vi "Open scan DB HOR.vi"(0 "dup path":path, 5 "Bytes":i64, 7 "Crop top":i32, 9 "Crop bottom":dbl, 11 "Start wavelength":dbl, 12 "End wavelength":dbl, 13 "gap":i32) -> (3 "Bytes done":i64, 4 "Intensity":sgl[](array[numeric]), 15 "wavelengths":sgl[](array[numeric]))   [LabVIEW 2014]
panel:
  # "I havn't a clue \nwhy I thought\nI needed this\nbut it breaks if\nI take it away"
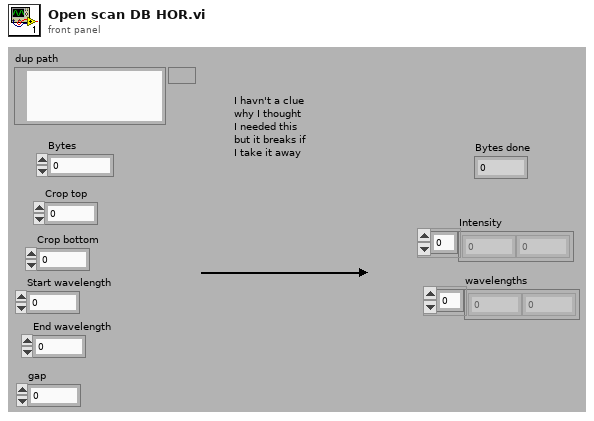
[diagram p1: front panel]
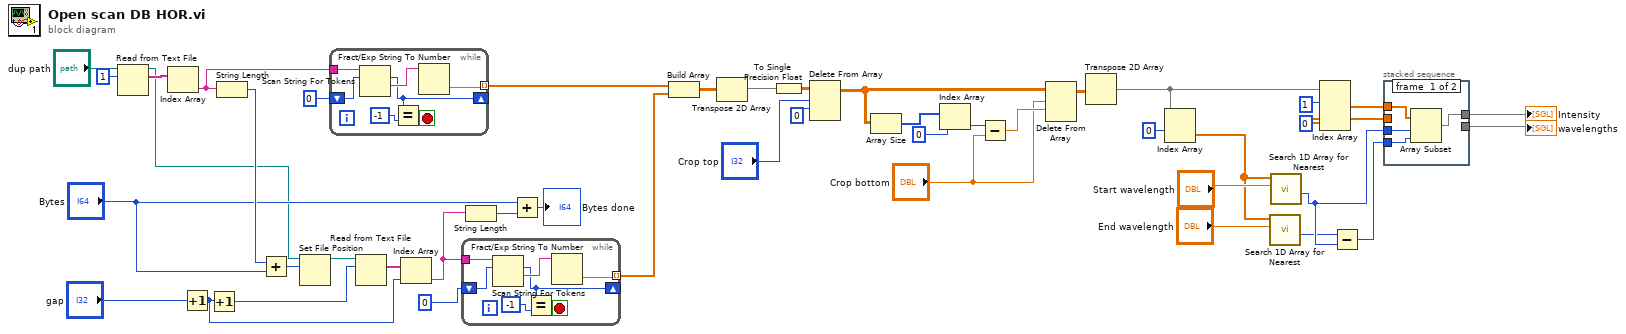
[diagram p0: block diagram]
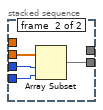
[diagram p2: hidden frame]
diagram:
  n1 = Read from Text File(file (use dialog)="dup path", count=1) -> (refnum out=w2:refnum<file>, text=w17:string[])  [unwired: 2 in, 2 out]
  n2 = Index Array(array=w17) -> (element=w1:string)  [unwired: 1 in]
  n3 = Increment(x="gap") -> (x+1=w8:i32)
  n4 = Increment(x=w8) -> (x+1=w9:i32)
  n5 = String Length(string=w1) -> (length=w14:i32)
  n6 = Add(x=w14, y="Bytes") -> (x+y=w15:i64)
  n7 = Set File Position(offset (in bytes) (0)=w15, refnum=w2) -> (refnum out=w24:refnum<file>)  [unwired: 2 in, 1 out]
  n8 = while {
    tunnel: [w50] -> w21 mode=indexing
    shift-right: [w49] -> _
    shift-left: 0 -> [w53]
    tunnel: w1 -> [w48]
    stop <- w52 stop-if-true
    n9 = Scan String For Tokens(8:w53, 9:w48) -> (1:w51:string, 2:w49:i32)  [unwired: 4 in, 2 out]
    n10 = Equal?(x=w49, y=-1) -> (x = y?=w52:bool)
    n11 = Fract/Exp String To Number(string=w51) -> (number=w50:dbl)  [unwired: 3 in, 1 out]
  }
  n12 = Read from Text File(file (use dialog)=w24, count=w9) -> (text=w20:string[])  [unwired: 2 in, 3 out]
  n13 = Index Array(array=w20, index=w8) -> (element=w23:string)
  n14 = while {
    tunnel: [w57] -> w22 mode=indexing
    shift-right: [w55] -> _
    shift-left: 0 -> [w60]
    tunnel: w23 -> [w56]
    stop <- w59 stop-if-true
    n15 = Scan String For Tokens(8:w60, 9:w56) -> (1:w58:string, 2:w55:i32)  [unwired: 4 in, 2 out]
    n16 = Equal?(x=w55, y=-1) -> (x = y?=w59:bool)
    n17 = Fract/Exp String To Number(string=w58) -> (number=w57:dbl)  [unwired: 3 in, 1 out]
  }
  n18 = String Length(string=w23) -> (length=w11:i32)
  n19 = Add(x="Bytes", y=w11) -> (x+y=→"Bytes done":i64)
  n20 = Build Array(w21, w22) -> (w26:dbl[][])
  n21 = Transpose 2D Array(2D array=w26) -> (transposed array=w27:dbl[][])
  n22 = To Single Precision Float(number=w27) -> (single precision float=w43:sgl[][])
  n23 = Delete From Array(array=w43, length="Crop top", index (row)=0) -> (array with subset deleted=w30:sgl[][])  [unwired: 1 in, 1 out]
  n24 = Array Size(array=w30) -> (size(s)=w34:i32[])
  n25 = Index Array(array=w34, index=0) -> (element=w31:i32)
  n26 = Subtract(x=w31, y="Crop bottom") -> (x-y=w32:dbl)
  n27 = Delete From Array(array=w30, length="Crop bottom", index (row)=w32) -> (array with subset deleted=w35:sgl[][])  [unwired: 1 in, 1 out]
  n28 = Transpose 2D Array(2D array=w35) -> (transposed array=w44:sgl[][])
  n29 = Index Array(array=w44, index (row)=0) -> (element=w5:sgl[])  [unwired: 1 in]
  n30 = call "Search 1D Array for Nearest.vi"("desired element"="End wavelength", "1D Array"=w5) -> ("closest index"=w3:i32)  [unwired: 8 in, 1 out]
  n31 = call "Search 1D Array for Nearest.vi"("desired element"="Start wavelength", "1D Array"=w5) -> ("closest index"=w6:i32)  [unwired: 8 in, 1 out]
  n32 = Index Array(array=w44, index (row) #1=1 ("index (row)"), index (row) #2=0 ("index (row)")) -> (element #1=w40:sgl[], element #2=w41:sgl[])  [unwired: 2 in]
  n33 = Subtract(x=w3, y=w6) -> (x-y=w42:i32)
  n34 = stacked-sequence {
    tunnel: w40 -> [w64 _]
    tunnel: w6 -> [w63 w67]
    tunnel: w42 -> [w62 w66]
    tunnel: w41 -> [_ w68]
    tunnel: [_ w65] -> w46
    tunnel: [w61 _] -> w16
    frame #0 {
      n35 = Array Subset(array=w64, index=w63, length=w62) -> (w61:sgl[])
    }
    frame #1 {
      n36 = Array Subset(array=w68, index=w67, length=w66) -> (w65:sgl[])
    }
  }
  "wavelengths" <- w46
  "Intensity" <- w16
